vi "test.vi"() -> ()   [LabVIEW 2017]
panel:
  in  "숫자형 2":dbl
  in  "숫자형":dbl
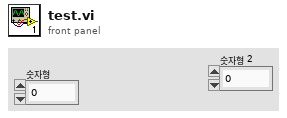
[diagram p1: front panel]
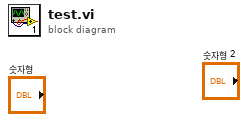
[diagram p0: block diagram]
diagram:
